vi "Check Size.vi"(0 "picture ref":refnum<vi>, 5 "State":T1={"Nspeakers"=13, "actions"=[], "Wspeaker"=13, "hover"={"type"=enum."None", "index"=0}, "locked"=FALSE, "states"=[], "sel speak"=13, "selected"=refnum, "Events"={"Selection change"=refnum}}) -> (6 "Min Control Width":i32, 8 "Min Control Height":i32)   [LabVIEW 2020, in "SAC Config.xctl"]
uses:
  SAC Config.xctl
  State.vi
  Hover Data.ctl
  Hover Item.ctl
  Speaker State.ctl
  Events.ctl
  Selection changed.ctl
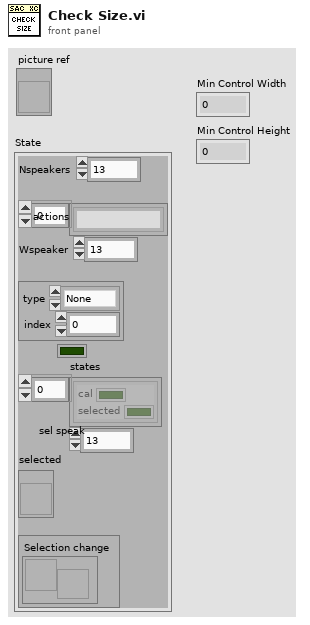
[diagram p1: front panel]
types:
  T1 = typedef "SAC Config.xctl/State.vi" = cluster{"Nspeakers":i32, "actions":string[], "Wspeaker":i32, "hover":T2, "locked":bool, "states":T4[], "sel speak":i32, "selected":refnum<vi>, "Events":T5}
  T2 = typedef "SAC Config.xctl/Hover Data.ctl" = cluster{"type":T3, "index":i32}
  T3 = typedef "SAC Config.xctl/Hover Item.ctl" = enum16{"None", "Speaker"}
  T4 = typedef "SAC Config.xctl/Speaker State.ctl" = cluster{"cal":bool, "selected":bool}
  T5 = typedef "SAC Config.xctl/Events.ctl" = cluster{"Selection change":refnum<user-event>}
  T6 = typedef "LVBoundsTypeDef.ctl" = cluster{"Width":u32, "Height":u32}
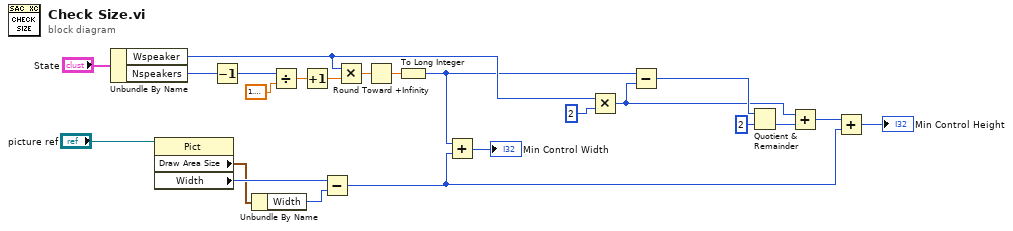
[diagram p0: block diagram]
diagram:
  n1 = Unbundle By Name("State") -> ("Wspeaker"=w15:i32, "Nspeakers"=w20:i32)
  n2 = property class="Pict"(reference="picture ref") -> ("Draw Area Size"=w12:T6, "Width"=w13:u32)  [unwired: 1 in, 2 out]
  n3 = Decrement(x=w20) -> (x-1=w19:i32)
  n4 = Unbundle By Name(w12) -> ("Width"=w14:u32)
  n5 = Divide(x=w19, y=1.5707963267948966) -> (x/y=w9:dbl)
  n6 = Increment(x=w9) -> (x+1=w8:dbl)
  n7 = Subtract(x=w13, y=w14) -> (x-y=w2:u32)
  n8 = Multiply(x=w15, y=w8) -> (x*y=w7:dbl)
  n9 = Round Toward +Infinity(x=w7) -> (ceil(x): smallest int >= x=w6:dbl)
  n10 = To Long Integer(number=w6) -> (32bit integer=w5:i32)
  n11 = Add(x=w5, y=w2) -> (x+y=→"Min Control Width":u32)
  n12 = Multiply(x=w15, y=2) -> (x*y=w16:i32)
  n13 = Subtract(x=w5, y=w16) -> (x-y=w18:i32)
  n14 = Quotient & Remainder(x=w18, y=2) -> (floor(x/y)=w22:i32)  [unwired: 1 out]
  n15 = Add(x=w16, y=w22) -> (x+y=w3:i32)
  n16 = Add(x=w3, y=w2) -> (x+y=→"Min Control Height":u32)
